vi "Get Control AttributeType.vi"(8 "error in (no error)":errorcluster, 11 "UIConfiguration in":refnum<class "UIConfiguration.lvclass">) -> (0 "error out":errorcluster, 2 "AttributeType":variant, 3 "UIConfiguration out":refnum<class "UIConfiguration.lvclass">)   [LabVIEW 2015, in "UIConfiguration.lvclass"]
uses:
  UIConfiguration.lvclass
  UIConfiguration.lvclass/UIConfiguration.ctl
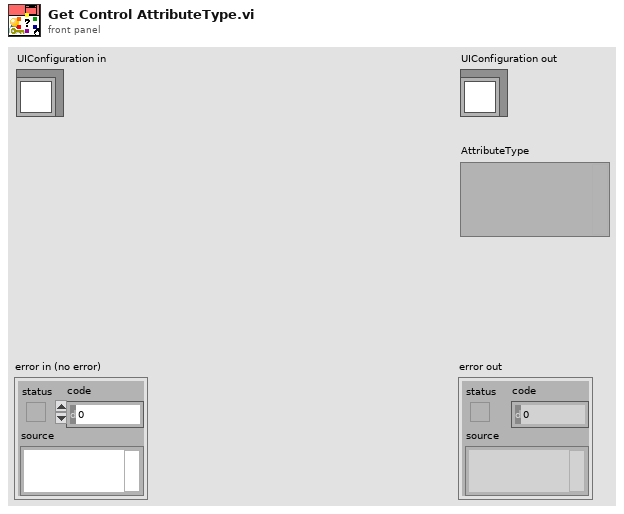
[diagram p1: front panel]
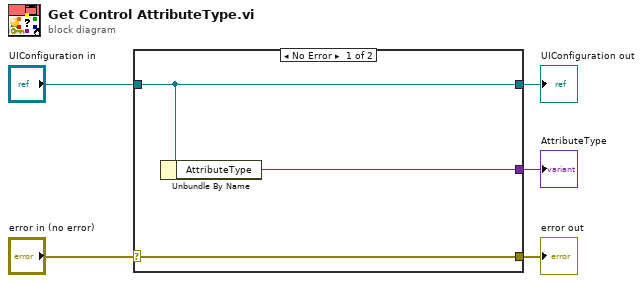
[diagram p0: block diagram]
diagram:
  n1 = case shown="No Error" "error in (no error)" {
    selector: "error in (no error)" -> [w8 w9]
    tunnel: [w8 w9] -> w4
    tunnel: [w7 w10] -> w2
    tunnel: "UIConfiguration in" -> [w7 w10]
    tunnel: [w6 _] -> w1
    frame No Error {
      n2 = Unbundle By Name(w7) -> ("AttributeType"=w6:variant)
    }
    frame Error {
    }
  }
  "error out" <- w4
  "UIConfiguration out" <- w2
  "AttributeType" <- w1
